vi "Create.vi"(8 "error in (no error)":errorcluster, 11 "ClientBase in":refnum<class "TCP.lvclass">) -> (0 "error out":errorcluster, 3 "ClientBase out":refnum<class "TCP.lvclass">)   [LabVIEW 2020, in "TCP.lvlib" / "TCP.lvclass"]
uses:
  TCP.lvclass
  TypeDefs/TCP Properties.ctl
  TCP.lvclass/TCP.ctl
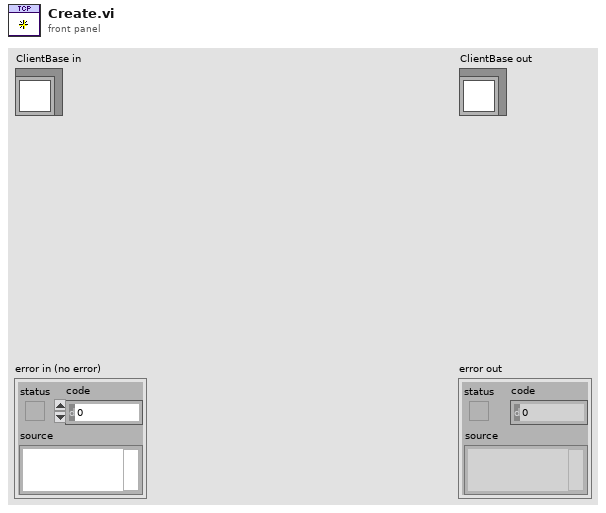
[diagram p1: front panel]
types:
  T1 = typedef "TCP.lvlib/TCP.lvclass/TCP Properties.ctl" = cluster{"Address":string, "Port":u16, "ID":string, "Connection ID":refnum<k5>, "Connected":bool, "Abort":bool}
  T2 = typedef "ConnectionProperties.ctl" = cluster{"Address":string, "Port":u16, "ID":string, "Connection ID":refnum<k5>, "Connected":bool, "Abort":bool}
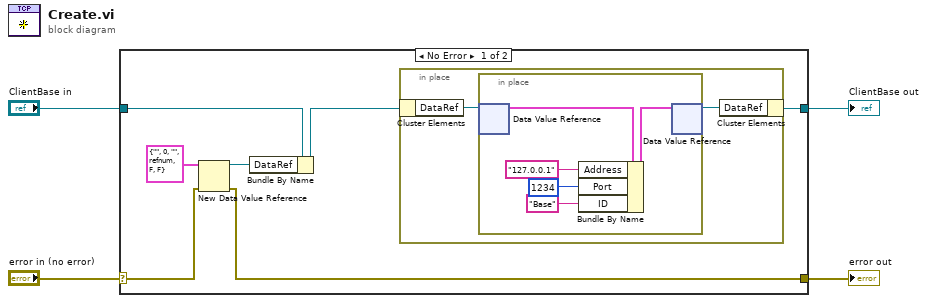
[diagram p0: block diagram]
diagram:
  n1 = case shown="No Error" "error in (no error)" {
    selector: "error in (no error)" -> [w7 w20]
    tunnel: [w6 w20] -> w3
    tunnel: [w5 w19] -> w1
    tunnel: "ClientBase in" -> [w11 w19]
    frame No Error {
      n2 = New Data Value Reference(data value=T1 {"Address"="", "Port"=0, "ID"="", "Connection ID"=refnum, "Connected"=FALSE, "Abort"=FALSE} ("ConnectionProperties"), error in=w7) -> (data value reference=w8:refnum<data-value>, error out=w6:errorcluster)
      n3 = Bundle By Name(cluster=w11, "DataRef"=w8) -> (w10:refnum<class "TCP.lvclass">)
      n4 = in-place {
        n5 = in-place-cluster #1(w10) -> ("DataRef"=w13:refnum<data-value>)
        n6 = in-place {
          n7 = in-place-dvr #2(w13) -> (w18:T2)  [unwired: 1 out]
          n8 = Bundle By Name(cluster=w18, "Address"="127.0.0.1", "Port"=u16 1234, "ID"="Base") -> (w17:T2)
          n9 = in-place-dvr #2(w17) -> (w12:refnum<data-value>)  [unwired: 1 out]
        }
        n10 = in-place-cluster #1("DataRef"=w12) -> (w5:refnum<class "TCP.lvclass">)
      }
    }
    frame Error {
    }
  }
  "error out" <- w3
  "ClientBase out" <- w1
